vi "AddCustomElement.vi"(8 "error in":errorcluster, 10 "Element":string, 11 "CustomData in":refnum<class "CustomData.lvclass">) -> (0 "error out":errorcluster, 2 "CustomElement":refnum<class "CustomElement.lvclass">, 3 "CustomData out":refnum<class "CustomData.lvclass">)   [LabVIEW 2021, in "ProligentXMLGenerator.lvlib" / "CustomData.lvclass"]
doc: "Add a custom element.\n\nThis value will not be interpreted by the DIT. It can be used to store data that will be used by another system."
uses:
  CustomData.lvclass
  CustomData.lvclass/CustomData.ctl
  CustomElement/CustomElement.lvclass
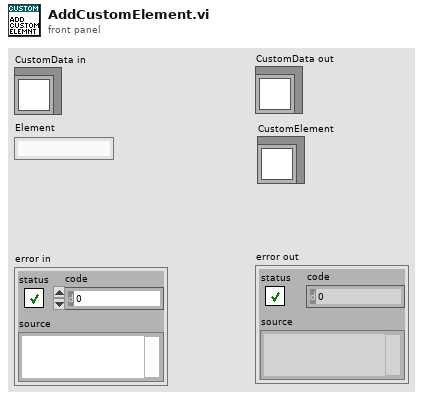
[diagram p1: front panel]
types:
  T1 = typedef "ProligentXMLGenerator.lvlib/CustomData.lvclass/Data.ctl" = cluster{"Name":string, "CustomElements":refnum<class "CustomElement.lvclass">[]}
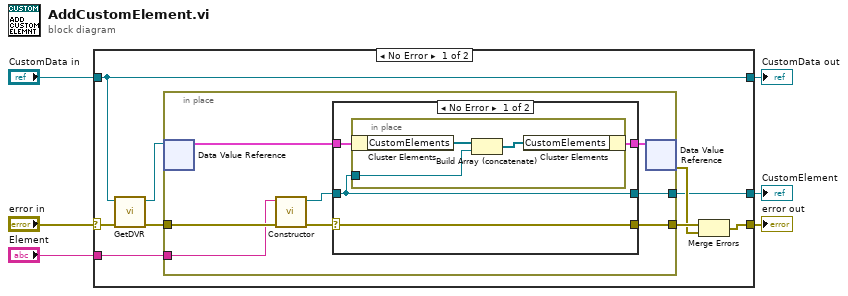
[diagram p0: block diagram]
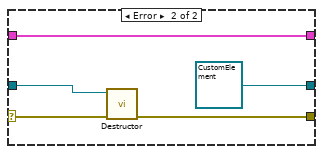
[diagram p2: hidden frame]
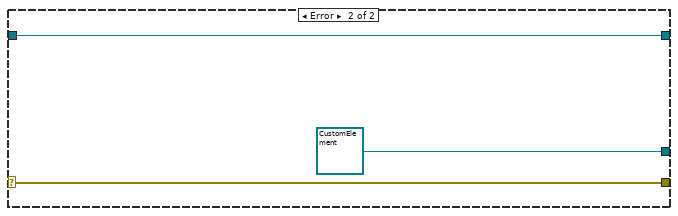
[diagram p3: hidden frame]
diagram:
  n1 = case shown="No Error" "error in" {
    selector: "error in" -> [w13 w38]
    tunnel: [w9 w38] -> w6
    tunnel: [w10 w37] -> w4
    tunnel: "CustomData in" -> [w10 w37]
    tunnel: "Element" -> [w15 _]
    tunnel: [w7 refnum<class "CustomElement.lvclass"> refnum ("ProligentResultProcessor:Any")] -> w1
    frame No Error {
      n2 = call "GetDVR.vi"("error in"=w13, "CustomDataType"=w10) -> ("error out"=w12:errorcluster, "DVRReference"=w11:refnum<data-value>)  [unwired: 8 in]
      n3 = in-place "In Place Element Structure" {
        in-place-border: w15 -> [w16]
        in-place-border: [w22] -> w14
        in-place-border: w12 -> [w21]
        in-place-border: [w18] -> w7
        n4 = in-place-dvr #1(w11) -> (w20:T1)  [unwired: 1 out]
        n5 = call "Constructor.vi"("error in"=w21, "Value"=w16) -> ("error out"=w23:errorcluster, "CustomElement"=w17:refnum<class "CustomElement.lvclass">)  [unwired: 8 in]
        n6 = case shown="No Error" w23 {
          selector: w23 -> [w27 w33]
          tunnel: [w24 w35] -> w19
          tunnel: [w27 w32] -> w22
          tunnel: w17 -> [w26 w34]
          tunnel: w20 -> [w25 w35]
          tunnel: [w26 refnum<class "CustomElement.lvclass"> refnum ("ProligentResultProcessor:Any")] -> w18
          frame No Error {
            n7 = in-place "In Place Element Structure" {
              in-place-border: w26 -> [w30]
              n8 = in-place-cluster #2(w25) -> ("CustomElements"=w29:refnum<class "CustomElement.lvclass">[])
              n9 = Build Array (concatenate)(w29, w30) -> (w28:refnum<class "CustomElement.lvclass">[])
              n10 = in-place-cluster #2("CustomElements"=w28) -> (w24:T1)
            }
          }
          frame Error {
            n11 = call "Destructor.vi"("error in"=w33, "CustomElement"=w34) -> ("error out"=w32:errorcluster)  [unwired: 9 in]
          }
        }
        n12 = in-place-dvr #1(w19) -> (w8:errorcluster)  [unwired: 1 out]
      }
      n13 = Merge Errors(w14, w8) -> (w9:errorcluster)
    }
    frame Error {
    }
  }
  "error out" <- w6
  "CustomData out" <- w4
  "CustomElement" <- w1
